vi "SummaryGui.vi"(11 "SeqData":T1={"BeginTS"=timestamp(0 s since 1904-01-01), "EndTS"=timestamp(0 s since 1904-01-01), "State"=enum."Init", "Status.Work"=enum."-", "Status.Process"=enum."-", "Status.Home"=enum."-", "Status.Wabco"=enum."-", "Status.Client"=enum."-", "BreakReason"=enum."-", "BreakSource"=enum."-", "DoorLock"=FALSE, "Status.Prod"=[], "UserAction"={"Stop"=FALSE, "Pause"=FALSE, "Next"=FALSE}, "UserData"={"GuiMode"=enum."Process", "Test"={"IgnoreResults"=FALSE, "IgnoreImages"=FALSE, "ServiceMode"=FALSE}, "ContinueOrder"=FALSE}, "Error"={"status"=FALSE, "code"=0, "source"=""}, "Code"={"Ready"=FALSE, "DoubleOrder"=FALSE, "OrderDone"=FALSE, "AllowSingleSlot"=FALSE, "CheckDM"=FALSE, "ThresholdA"=0, "ThresholdB"=0, "Plate"=enum."Wabco", "ImgPath"=path "", "Variant"={"State"=enum."Init", "ImgPath"=path "", "WabcoPlate"="", "WabcoProduct"="", "ClientProduct"="", "ClientPlate"="", "TotalQuantity"=0, "OrderQuantity"=0, "Serial"=0, "Wabco"={"LaserJob"="", "AdditionalTxt"="037", "FactoryCode"="", "RevID"=0, "ForkID"=0, "FailuresLimit"=0, "GlobalCnt"=0, "Bank"=0, "SerialFormat"=enum."6 dig", "CoordA"={"X"=0.0, "Y"=0.0, "Angle"=0.0}, "CoordB"={"X"=0.0, "Y"=0.0, "Angle"=0.0}, "DMCconfig"=0}, "Client"={"LaserJob"="", "AdditionalTxt"="", "FactoryCode"="037", "RevID"=0, "ForkID"=0, "FailuresLimit"=0, "GlobalCnt"=0, "Bank"=0, "SerialFormat"=enum."6 dig", "CoordA"={"X"=0.0, "Y"=0.0, "Angle"=0.0}, "CoordB"={"X"=0.0, "Y"=0.0, "Angle"=0.0}, "DMCconfig"=0}}}, "Rotations"=0, "ProdIdx"=0, "ProdDone"=[], "PrintedSerials-Wabco"=[], "PrintedSerials-Client"=[], "Counters-Wabco"={"Expected"=0, "Done"=0, "OK"=0, "NOK"=0, "NOKlimit"=0, "Part"=0, "PartOK"=0}, "Counters-Client"={"Expected"=0, "Done"=0, "OK"=0, "NOK"=0, "NOKlimit"=0, "Part"=0, "PartOK"=0}}) -> ()   [LabVIEW 2016]
uses:
  Sequence/Sequence.Data.ctl
  Sequence/Sequence.State.ctl
  Sequence/Sequence.Step.Status.ctl
  Sequence/Sequence.Test.BreakReason.ctl
  Sequence/Sequence.Test.BreakSource.ctl
  Sequence/Sequence.Test.Status.ctl
  Sequence/Sequence.Slot.StatusData.ctl
  Sequence/Sequence.Test.Unload.Status.ctl
  Sequence/Sequence.Prod.StatusData.ctl
  Sequence/Sequence.UserActions.ctl
  Sequence/Sequence.UserData.ctl
  Sequence/Sequence.MainMode.ctl
  MainGui.TestOptions.ctl
  Sequence/Sequence.Code.Sets.ctl
  Sequence/Sequence.PlateType.ctl
  Logger/Logger.Variant.Sets.ctl
  Station/Station.Changeover.State.vi
  Station/Station.Plate.Properties.ctl
  Sequence/Sequence.Code.SerialFormat.ctl
  Drivers/V7310/LowLevel/V7310.Job.Sets.ctl
  Sequence/Sequence.Counters.ctl
  SummaryGui.Action.ctl
  tools/Translator/Translator.Message.ctl
  tools/Translator/Translator.FormatMessage.vi
  Global/ApplicationGlobal.vi
  tools/Translator/Translator.Global.vi
panel:
  out "container removed":bool
  in  "WabcoPlateSelect":bool
  in  "ClientPlateSelect":bool
  out "Total 2":u16 caption="Wymagane"
  out "NOK 2":u16 caption="NOK"
  out "OK 2":u16 caption="OK"
  out "Done 2":u16 caption="Zrobione"
  out "Total":u16 caption="Wymagane"
  out "NOK":u16
  out "OK":u16
  out "Done":u16 caption="Zrobione"
  out "ClientPlate":picture
  out "Client Plate Status":string caption="Status tabliczki Klienta"
  out "WabcoPlate":picture
  out "Wabco Plate Status":string caption="Status tabliczki Wabco"
  out "Message":string
  in  "OKButton":bool
  out "_loop":i32(ring)=4
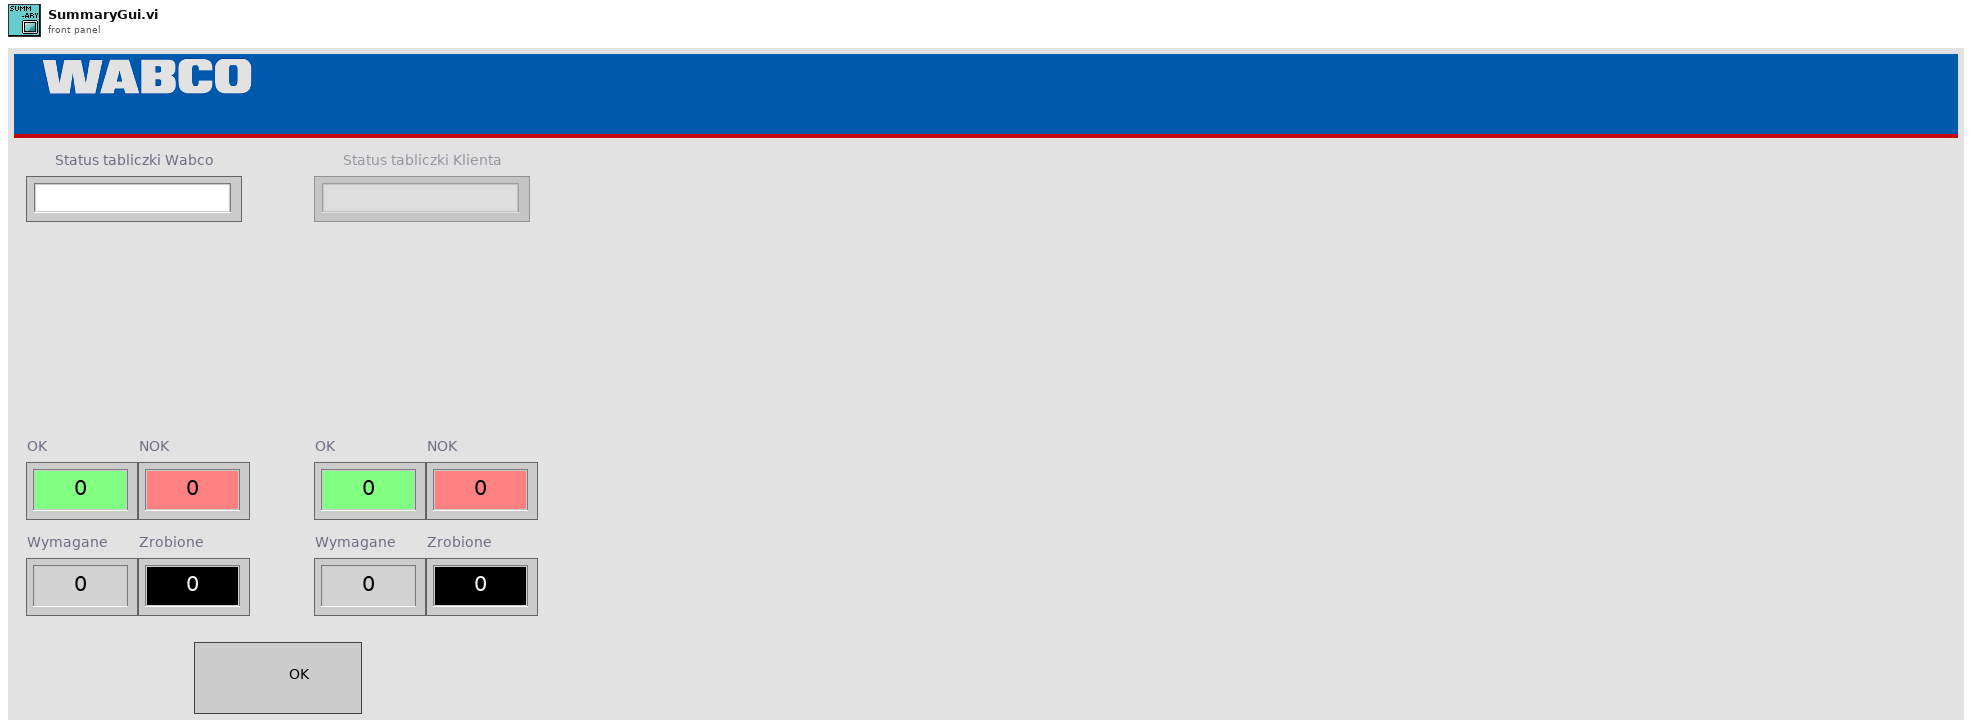
[diagram p1: front panel]
types:
  T1 = typedef "Sequence.Data.ctl" = cluster{"BeginTS":timestamp, "EndTS":timestamp, "State":T2, "Status.Work":T3, "Status.Process":T3, "Status.Home":T3, "Status.Wabco":T3, "Status.Client":T3, "BreakReason":T4, "BreakSource":T5, "DoorLock":bool, "Status.Prod":T6[], "UserAction":T10, "UserData":T11, "Error":errorcluster, "Code":T14, "Rotations":i32, "ProdIdx":i32, "ProdDone":T6[], "PrintedSerials-Wabco":i32[], "PrintedSerials-Client":i32[], "Counters-Wabco":T21, "Counters-Client":T21}
  T2 = typedef "Sequence.State.ctl" = enum16{"Init", "Idle", "Home", "Work", "Run", "Pause"}
  T3 = typedef "Sequence.Step.Status.ctl" = enum16{"-", "Pending", "Running", "Skipped", "Passed", "Failed", "Done", "Error", "Aborted", "Stopped"}
  T4 = typedef "Sequence.Test.BreakReason.ctl" = enum16{"-", "NOK container", "OK container", "Rev empty", "Rev missing", "Rev wrong", "Fork missing", "Fork wrong", "NOK limit", "Unload failure", "Single slot", "Part done", "Err: Prod move work", "Err: Prod move home", "Err: Prod lift work", "Err: Prod lift home", "Err: Prod Arm Work", "Err: Prod Arm NOK", "Err: Prod Arm OK", "Err: Prod NOK suck", "Err: Prod NOK drop", "Err: Prod OK missing", "Err: Prod OK suck", "Err: Prod OK drop"}
  T5 = typedef "Sequence.Test.BreakSource.ctl" = enum16{"-", "A", "B", "A/B"}
  T6 = typedef "Sequence.Test.Status.ctl" = cluster{"Slot":T7, "A":T9, "B":T9}
  T7 = typedef "Sequence.Slot.StatusData.ctl" = cluster{"ID":i32, "Unload":T8, "TS":timestamp, "duration":u32}
  T8 = typedef "Sequence.Test.Unload.Status.ctl" = enum16{"init", "check NOK", "check OK", "wait on NOK", "wait on OK", "wait on Unload", "done"}
  T9 = typedef "Sequence.Prod.StatusData.ctl" = cluster{"status":T3, "pause":T4, "present":bool, "printed":bool, "scanned":bool, "tuned":bool, "removed":bool, "LaserVariables":string[], "ScanerReadOut":string, "path":path, "corners":cluster{"X":i32, "Y":i32}[], "verification":u8}
  T10 = typedef "Sequence.UserActions.ctl" = cluster{"Stop":bool, "Pause":bool, "Next":bool}
  T11 = typedef "Sequence.UserData.ctl" = cluster{"GuiMode":T12, "Test":T13, "ContinueOrder":bool}
  T12 = typedef "Sequence.MainMode.ctl" = enum16{"Process", "Base", "Order", "Manual", "Logs", "Results", "Stats", "DMC Config"}
  T13 = typedef "MainGui.TestOptions.ctl" = cluster{"IgnoreResults":bool, "IgnoreImages":bool, "ServiceMode":bool}
  T14 = typedef "Sequence.Code.Sets.ctl" = cluster{"Ready":bool, "DoubleOrder":bool, "OrderDone":bool, "AllowSingleSlot":bool, "CheckDM":bool, "ThresholdA":u8, "ThresholdB":u8, "Plate":T15, "ImgPath":path, "Variant":T16}
  T15 = typedef "Sequence.PlateType.ctl" = enum16{"Wabco", "Client"}
  T16 = typedef "Logger.Variant.Sets.ctl" = cluster{"State":T17, "ImgPath":path, "WabcoPlate":string, "WabcoProduct":string, "ClientProduct":string, "ClientPlate":string, "TotalQuantity":u16, "OrderQuantity":u16, "Serial":i32, "Wabco":T18, "Client":T18}
  T17 = typedef "Station.Changeover.State.vi" = enum16{"Init", "Scaning", "NOK", "Wait for ack", "Ready"}
  T18 = typedef "Station.Plate.Properties.ctl" = cluster{"LaserJob":string, "AdditionalTxt":string, "FactoryCode":string, "RevID":u8, "ForkID":u8, "FailuresLimit":u16, "GlobalCnt":i32, "Bank":u8, "SerialFormat":T19, "CoordA":T20, "CoordB":T20, "DMCconfig":i32}
  T19 = typedef "Sequence.Code.SerialFormat.ctl" = enum8{"", "6 dig", "7 dig"}
  T20 = typedef "V7310.Job.Sets.ctl" = cluster{"X":dbl, "Y":dbl, "Angle":dbl}
  T21 = typedef "Sequence.Counters.ctl" = cluster{"Expected":u16, "Done":u16, "OK":u16, "NOK":u16, "NOKlimit":u16, "Part":u16, "PartOK":u16}
  T22 = typedef "SummaryGui.Action.ctl" = enum32{"idle", "constructor", "destructor", "--- SummaryGUI ---", "wait for container"}
  T23 = enum8{"Enabled", "Disabled", "Disabled and Grayed Out"}
  T24 = typedef "Translator.Message.ctl" = enum16{"-", "Event confirmed", "Log out", "Log in", "Shutdown", "Cancel", "Start", "Begin time", "End time", "Duration", "Service Mode", "Ignore Results", "Serial Format", "On", "Off", "OK", "NOK", "NOK %s", "Home", "Work", "Close", "Open", "In progress...", "Missing", "Empty", "Hardware failure", "Initial", "Default", "Total", "Out of range", "Free disk space is below 1GB - contact technician", "Error %d >> %s", "Error %d >> %s >> %s", "Msg %d >> %s", "Laser msg %d %s", "Laser cmd error %s %d", "Laser cmd failed %s", "Laser cmd warning %s", "Laser disconnected", "Laser status %s", "Laser already started", "Laser job unkonwn %s", "Laser job missing %s", "Laser job select failure %s", "Unable to start laser printing (%s)", "Unable to stop laser printing (%s)", "Laser marking aborted", "Laser marking timeout", "Unable to reset Laser Interlock (%s)", "Unable to trigger Laser. Laser not ready (%s)", "Laser job '%s' coordinates not configured", "Starting %s", "Quitting %s", "Configured", "Initializing", "Quitting", "Loading", "Loaded %d results", "Loaded %d events", "Running", "Stopped", "Summary", "Laser", "Do you want to continue?", "Do you want to delete the configuration?", "The configuration is being used by an order. Unable to delete!", "Press confirm button", "Station is not based. Do you want to exit?", "Station requires changeover. Do you want to run the test?", "Test options are not set as default. Do you want to continue?", "Formatting of WabcoNo is disabled. Do you want to continue?", "Product not detected. Do you want to continue?", "Product scan failed. Do you want to continue?", "Calibration", "Log out?", "System", "All", "IDLE", "Translating...%s", "Not found", "Alarm %s", "Run", "Skip", "Abort", "Repeat", "Please wait...", "Database disconnected", "Database disconnected - changeover disabled!", "Login to database successful", "Login to database failed: %d; %s", "Unable to check the product status of reference %d - database disconnected", "Unable to set the product status of reference %d - database disconnected", "Variant file backup %s", "Read variant (%s)", "Result", "Station armed!", "Station requires changeover!", "Select reference number...", "EMERGENCY BUTTON - press Control button", "EMERGENCY DOOR - press Control button", "Resetting Emergency...", "Unable to reset safety circuit - Emergency Button pressed", "Unable to reset safety circuit - Emergency Side Door open", "Station not based", "Station based", "Station not empty", "Station basing...", "No order", "Press Start to begin new order", "Scanning new order", "Order NOK. Correct or scan again", "Order OK. Press Accept", "Order ready", "Revolver incorrect", "Fork incorrect", "Revolver missing", "Revolver empty", "Container missing", "Offline results", "Offline statistics", "Updating statistics %.1f %%", "DMC Configurator", "Door open", "Close the front door", "Press start button", "Done. Open the front door", "Running...", "Running...%.1f %%", "Pause %s", "Pause %s. NOK container missing", "Pause %s. OK container missing", "Pause %s. Revolver empty", "Pause %s. Revolver missing", "Pause %s. Revolver incorrect", "Pause %s. Fork missing", "Pause %s. Fork incorrect", "Pause %s. Too many failures", "Pause %s. Unloading failure", "Pause %s. One slot is not working", "Pause %s. Part order is done. Empty OK container", "Pause %s. Unable to move product to slot", "Pause %s. Unable to move back product pusher", "Pause %s. Unable to lift product", "Pause %s. Unable to move back product lifter", "Pause %s. Unable to move product arm to Work", "Pause %s. Unable to move product arm to NOK", "Pause %s. Unable to move product arm to OK", "Pause %s. Unable to unsuck the NOK product", "Pause %s. Unable to drop the NOK product", "Pause %s. Product OK missing", "Pause %s. Unable to unsuck the OK product", "Pause %s. Unable to drop the OK product", "Stopping...", "File '%s' is missing", "File '%s' is broken", "File '%s' is running", "Log file started (%s)", "Log file ended (%s)", "Log file stopped (%s)", "Log file ignored (%s)", "Log file exported (%s)", "Log file export failed (%s)", "Wrong serial number in log file", "Wrong reference number in log file", "Test steps are missing", "%s = %.3f", "Process param '%s' not found in DB", "Process param '%s' wrong order", "Process param '%s' value %.3f out of limits (%.3f; %.3f)", "Step%d param '%s' not found in DB", "Step%d param '%s' wrong order", "Step%d param '%s' value %.3f out of limits (%.3f; %.3f)", "Step%d EV '%s' not found in DB", "Step%d EV '%s' wrong order", "\"%s\" not found in DB", "\"%s\" wrong order", "\"%s\" value %.3f out of limits (%.3f; %.3f)", "\"%s\" not found in software", "Process init (%s)", "Process started", "Process restarted", "Process run", "Process done", "Process done - remove OK container", "Process aborted", "Process aborted at work", "Process aborted at home", "Process error", "Process error at home", "Process error at work", "Process close", "Process pause", "Process continue", "Process door open", "Process door close", "Process pause at slot %s due to %s", "Select plate from the order to process", "Do you want to start the process?", "Do you want to continue the process?", "There is unfinished order. Do you want to put the new order?", "Product %s %d OK", "Product %s %d NOK", "Unable to unload the slot %s. Product missing in the slot", "Unable to unload the slot %s. Product already in the arm", "Unable to accept the product as OK. Product missing in slot %s", "Unable to accept the product as OK. Product could not drop into the container at slot %s", "Unable to accept the product as NOK. Product could not drop into the container at slot %s", "Scan failed. Error %s", "Scan failed. Scanner disconnected", "Scan failed. Wrong Wabco number %d, limit (%d,%d)", "Scan failed. Wrong serial number %d, limit (%d,%d)", "Scan failed. Wrong date %d, limit (%d,%d)", "Scan failed. Wrong product wabco number %d (expected %d)", "Scan failed. Wrong product serial number %d (expected > 0)", "Scan OK %s", "Scan failed. Unable to determine table position (%s)", "Scan failed. Timeout", "Tune failed. Scanner disconnected", "Tune failed. Timeout", "%s = %d", "%s = %d->%d", "Unable to set %s = %.2f - Air Pressure Inside off", "Unable to set digital output '%s' = %d", "Unable to activate air pressure inside - timeout", "Unable to activate air pressure inside - aborted", "Unable to switch on Air Main Valve - Air Pressure Inlet off", "Unable to switch on Air Main Valve - Door open", "Unable to switch off Air Main Valve - timeout", "Unable to switch off Air Main Valve - aborted", "Unable to rotate Table - timeout", "Unable to rotate Table - aborted", "Unable to rotate Table - Product Move not in Home position", "Unable to rotate Table - Air Pressure Inside off", "Unable to rotate Table - Product Lift A not in Home position", "Unable to rotate Table - Product Lift B not in Home position", "Unable to rotate Table - unlock before movement timeout", "Unable to rotate Table - lock after movement timeout", "Unable to move Table Lock to %s position - timeout", "Unable to move Table Lock to %s position - aborted", "Unable to move Table Lock to %s position - Air Pressure Inside off", "Unable to move Table Lock to %s position - Table not in position", "Unable to move Product Lift A to %s position - timeout", "Unable to move Product Lift B to %s position - timeout", "Unable to move Product Lift A to %s position - aborted", "Unable to move Product Lift B to %s position - aborted", "Unable to move Product Lift A to %s position - Air Pressure Inside off", "Unable to move Product Lift B to %s position - Air Pressure Inside off", "Unable to move Product Lift A to %s position - Table not locked", "Unable to move Product Lift B to %s position - Table not locked", "Unable to move Product Lift A to %s position - Product Arm not in Work position", "Unable to move Product Lift B to %s position - Product Arm not in Work position", "Unable to set Product Suction Gripper %s to %s - timeout", "Unable to set Product Suction Gripper %s to %s - aborted", "Unable to set Product Suction Gripper %s to %s - Air Pressure Inside off", "Unable to set Product Suction Gripper %s to %s - Table slot unkown", "Unable to move Product Arm to %s position - timeout", "Unable to move Product Arm to %s position - aborted", "Unable to move Product Arm to %s position - Air Pressure Inside off", "Unable to move Product Arm to %s position - Product Lift A not in Home position", "Unable to move Product Arm to %s position - Product Lift B not in Home position", "Unable to move Product to %s position - timeout", "Unable to move Product to %s position - aborted", "Unable to move Product to %s position - Air Pressure Inside off", "Unable to move Product to %s position - Table not in position"}
  T25 = typedef "FestoCPX.Station.ButtonsState.ctl" = cluster{"Start":bool, "Stop":bool, "Control":bool}
  T26 = typedef "LVPositionTypeDef.ctl" = cluster{"Left":i32, "Top":i32}
  T27 = typedef "imagedata.ctl" = cluster{"image type":i32, "image depth":i32, "image":u8[], "mask":u8[], "colors":u32[], "Rectangle":cluster{"left":i16, "top":i16, "right":i16, "bottom":i16}}
  T28 = typedef "FestoCPX.Station.ProdPresent.ctl" = cluster{"Slot1":cluster{"A":bool, "B":bool}, "Slot2":cluster{"A":bool, "B":bool}, "Slot3":cluster{"A":bool, "B":bool}, "Slot4":cluster{"A":bool, "B":bool}, "Final":cluster{"A":bool, "B":bool}, "OK":cluster{"A":bool, "B":bool}, "Container":cluster{"OK":bool, "NOK":bool}}
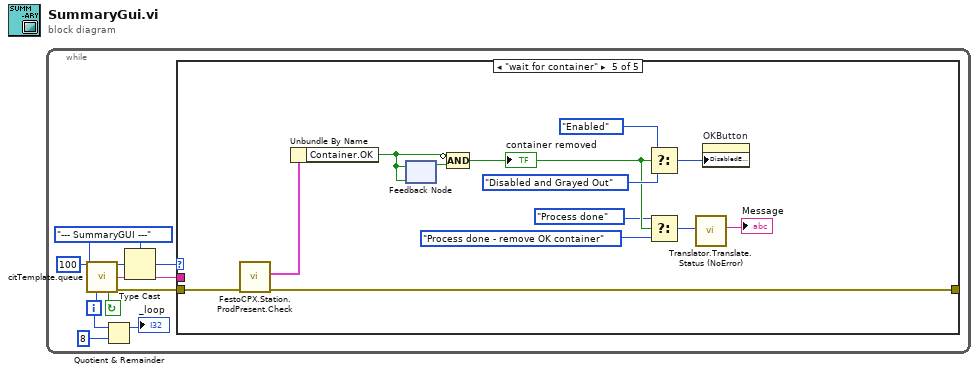
[diagram p0: block diagram]
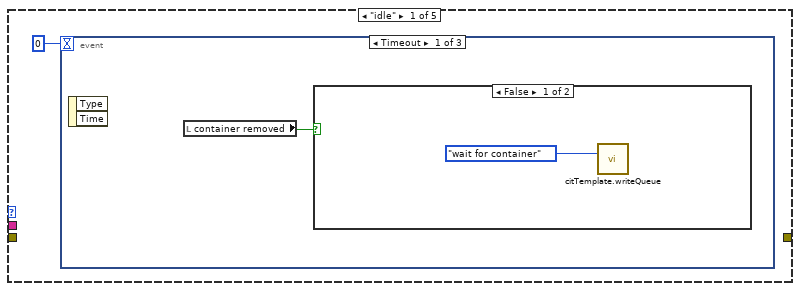
[diagram p2: hidden frame]
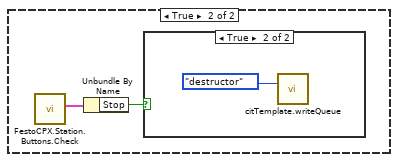
[diagram p3: hidden frame]
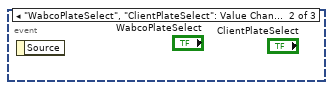
[diagram p5: hidden frame]
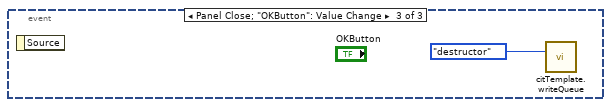
[diagram p6: hidden frame]
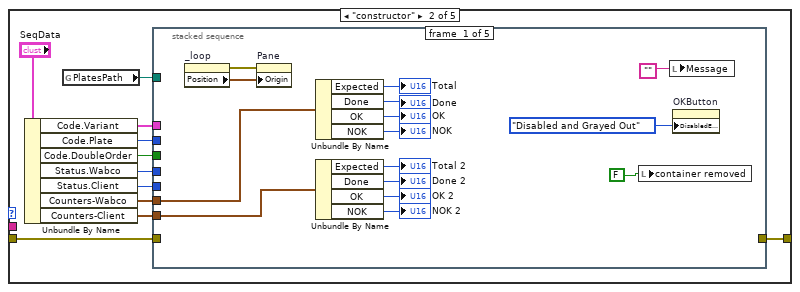
[diagram p7: hidden frame]
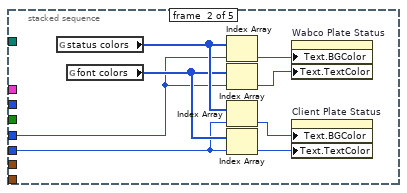
[diagram p8: hidden frame]
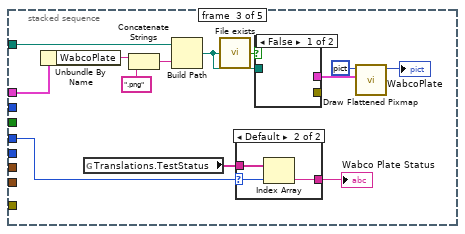
[diagram p9: hidden frame]
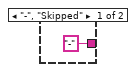
[diagram p10: hidden frame]
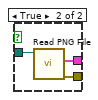
[diagram p11: hidden frame]
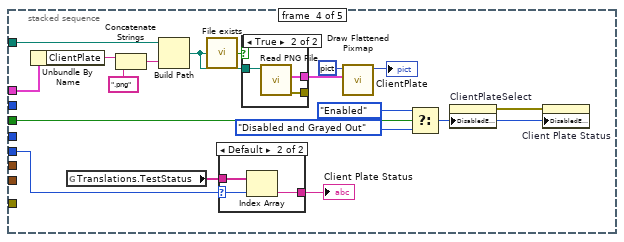
[diagram p12: hidden frame]
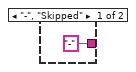
[diagram p13: hidden frame]
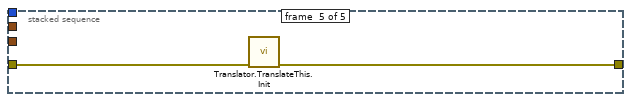
[diagram p15: hidden frame]
diagram:
  n1 = while {
    i -> [w1]
    stop <- w10 continue-if-true
    w4 = SummaryGui.Action."--- SummaryGUI ---" ("Action")
    n2 = call "citTemplate.queue.vi"("ms timeout (250 ms)"=100, "event enum"=w4, "iteration (-1)"=w1) -> ("event out"=w8:u32, "(flatten) data out"=w5:string, "continue"=w10:bool, "error out"=w6:errorcluster)  [unwired: 2 in, 7 out]
    n3 = Quotient & Remainder(x=w1, y=8) -> (x-y*floor(x/y)=→"_loop":i32)  [unwired: 1 out]
    n4 = Type Cast(type=w4, x=w8) -> (*(type *) &x=w7:T22)
    n5 = case shown="\"wait for container\"" w7 {
      tunnel: w6 -> [_ w22 _ _ w109]
      tunnel: w5 -> [_ _ _ _ _]
      tunnel: [_ w21 _ _ w108] -> _
      frame "idle" {
        n6 = event shown="[0] Timeout" {
          selector: _ -> [_ _ _]
          dyn-events: _ -> [_ _ _]
          timeout: 0 -> [_ _ _]
          event Timeout {
            n7 = event-data() -> ()  [unwired: 3 out]
            n8 = local read "container removed"() -> (w12:bool)
            n9 = case shown="False" w12 {
              frame False {
                n10 = call "citTemplate.writeQueue.vi"("event in (if not connected:all statemachine with data event)"=SummaryGui.Action."wait for container" ("Action")) -> ()  [unwired: 14 in, 1 out]
              }
              frame True {
                n11 = call "FestoCPX.Station.Buttons.Check.vi"() -> ("Buttons.State"=w15:T25)  [unwired: 10 in, 1 out]
                n12 = Unbundle By Name(w15) -> ("Stop"=w14:bool)
                n13 = case shown="True" w14 {
                  frame False {
                  }
                  frame True {
                    n14 = call "citTemplate.writeQueue.vi"("event in (if not connected:all statemachine with data event)"=SummaryGui.Action."destructor" ("Action")) -> ()  [unwired: 14 in, 1 out]
                  }
                }
              }
            }
          }
          event "WabcoPlateSelect", "ClientPlateSelect": Value Change {
            n15 = event-data() -> ()  [unwired: 2 out]
          }
          event Panel Close; "OKButton": Value Change {
            n16 = event-data() -> ()  [unwired: 2 out]
            n17 = call "citTemplate.writeQueue.vi"("event in (if not connected:all statemachine with data event)"=SummaryGui.Action."destructor" ("Action")) -> ()  [unwired: 14 in, 1 out]
          }
        }
      }
      frame "constructor" {
        n18 = Unbundle By Name("SeqData") -> ("Code.Variant"=w27:T16, "Code.Plate"=w26:T15, "Code.DoubleOrder"=w23:bool, "Status.Wabco"=w25:T3, "Status.Client"=w24:T3, "Counters-Wabco"=w20:T21, "Counters-Client"=w19:T21)
        n19 = global read "ApplicationGlobal.vi" "PlatesPath"() -> (w28:path)
        n20 = stacked-sequence {
          tunnel: w28 -> [_ _ w56 w82 _]
          tunnel: w27 -> [_ _ w52 w75 _]
          tunnel: w26 -> [_ _ _ _ _]
          tunnel: w25 -> [_ w49 w55 _ _]
          tunnel: w24 -> [_ w46 _ w74 _]
          tunnel: w23 -> [_ _ _ w76 _]
          tunnel: w22 -> [_ _ _ _ w98]
          tunnel: [_ _ _ _ w97] -> w21
          tunnel: w20 -> [w41 _ _ _ _]
          tunnel: w19 -> [w38 _ _ _ _]
          frame #0 {
            n21 = property on="_loop" class="Ring (strict)"() -> (error out=w32:errorcluster, "Position"=w33:T26)  [unwired: 2 in, 1 out]
            n22 = property on="Pane" class="Pane"(error in=w32, "Origin"=w33) -> ()  [unwired: 1 in, 2 out]
            n23 = Unbundle By Name(w41) -> ("Expected"=→"Total":u16, "Done"=→"Done":u16, "OK"=→"OK":u16, "NOK"=→"NOK":u16)
            n24 = Unbundle By Name(w38) -> ("Expected"=→"Total 2":u16, "Done"=→"Done 2":u16, "OK"=→"OK 2":u16, "NOK"=→"NOK 2":u16)
            n25 = local write "container removed"(FALSE ("container removed")) -> ()
            n26 = local write "Message"("") -> ()
            n27 = property on="OKButton" class="Bool"("DisabledEnum"=T23."Disabled and Grayed Out" ("Disabled")) -> ()  [unwired: 2 in, 2 out]
          }
          frame #1 {
            n28 = global read "ApplicationGlobal.vi" "status colors"() -> (w51:u32[])
            n29 = global read "ApplicationGlobal.vi" "font colors"() -> (w50:u32[])
            n30 = Index Array(array=w51, index=w49) -> (element=w48:u32)
            n31 = Index Array(array=w50, index=w49) -> (element=w47:u32)
            n32 = Index Array(array=w51, index=w46) -> (element=w45:u32)
            n33 = Index Array(array=w50, index=w46) -> (element=w44:u32)
            n34 = property on="Wabco Plate Status" class="Str"("Text.BGColor"=w48, "Text.TextColor"=w47) -> ()  [unwired: 2 in, 2 out]
            n35 = property on="Client Plate Status" class="Str"("Text.BGColor"=w45, "Text.TextColor"=w44) -> ()  [unwired: 2 in, 2 out]
          }
          frame #2 {
            n36 = Unbundle By Name(w52) -> ("WabcoPlate"=w61:string)
            n37 = global read "Translator.Global.vi" "Translations.TestStatus"() -> (w53:string[])
            n38 = Concatenate Strings(w61, ".png" ("string")) -> (w62:string)
            n39 = Build Path(base path=w56, name or relative path=w62) -> (appended path=w60:path)
            n40 = call "File exists.vi"("file path"=w60) -> ("exists?"=w59:bool)  [unwired: 4 in]
            n41 = case shown="Default" w55 {
              selector: w55 -> [_ w67]
              tunnel: ["-" ("String") w66] -> w54
              tunnel: w53 -> [_ w68]
              frame "-", "Skipped" {
              }
              frame Default {
                n42 = Index Array(array=w68, index=w67) -> (element=w66:string)
              }
            }
            "Wabco Plate Status" <- w54
            n43 = case shown="False" w59 {
              tunnel: w60 -> [_ w71]
              tunnel: [_ w70] -> w57
              tunnel: [_ w69] -> _
              frame False {
              }
              frame True {
                n44 = call <vilib>:"Read PNG File.vi"("path to PNG file"=w71) -> ("error out"=w69:errorcluster, "image data"=w70:T27)  [unwired: 8 in, 1 out]
              }
            }
            n45 = call <vilib>:"Draw Flattened Pixmap.vi"("image data"=w57, "picture"=picture data[5B]) -> ("new picture"=→"WabcoPlate":picture)  [unwired: 7 in]
          }
          frame #3 {
            n46 = Unbundle By Name(w75) -> ("ClientPlate"=w81:string)
            n47 = global read "Translator.Global.vi" "Translations.TestStatus"() -> (w73:string[])
            n48 = Concatenate Strings(w81, ".png" ("string")) -> (w87:string)
            n49 = Build Path(base path=w82, name or relative path=w87) -> (appended path=w86:path)
            n50 = call "File exists.vi"("file path"=w86) -> ("exists?"=w85:bool)  [unwired: 4 in]
            n51 = case shown="Default" w74 {
              selector: w74 -> [_ w92]
              tunnel: ["-" ("String") w91] -> w72
              tunnel: w73 -> [_ w93]
              frame "-", "Skipped" {
              }
              frame Default {
                n52 = Index Array(array=w93, index=w92) -> (element=w91:string)
              }
            }
            "Client Plate Status" <- w72
            n53 = case shown="True" w85 {
              tunnel: w86 -> [_ w96]
              tunnel: [_ w95] -> w83
              tunnel: [_ w94] -> _
              frame False {
              }
              frame True {
                n54 = call <vilib>:"Read PNG File.vi"("path to PNG file"=w96) -> ("error out"=w94:errorcluster, "image data"=w95:T27)  [unwired: 8 in, 1 out]
              }
            }
            n55 = call <vilib>:"Draw Flattened Pixmap.vi"("image data"=w83, "picture"=picture data[5B]) -> ("new picture"=→"ClientPlate":picture)  [unwired: 7 in]
            n56 = Select(t=T23."Enabled" ("Disabled"), s=w76, f=T23."Disabled and Grayed Out" ("Disabled")) -> (s? t:f=w78:T23)
            n57 = property on="ClientPlateSelect" class="Bool"("DisabledEnum"=w78) -> (error out=w77:errorcluster)  [unwired: 2 in, 1 out]
            n58 = property on="Client Plate Status" class="Str"(error in=w77, "DisabledEnum"=w78) -> ()  [unwired: 1 in, 2 out]
          }
          frame #4 {
            n59 = call "Translator.TranslateThis.Init.vi"("error in"=w98) -> ("error out"=w97:errorcluster)  [unwired: 10 in]
          }
        }
      }
      frame "destructor" {
      }
      frame "--- SummaryGUI ---" {
      }
      frame "wait for container" {
        n60 = call "FestoCPX.Station.ProdPresent.Check.vi"("error in"=w109) -> ("error out"=w108:errorcluster, "Prod Present"=w111:T28)  [unwired: 5 in, 4 out]
        n61 = Unbundle By Name(w111) -> ("Container.OK"=w99:bool)
        n62 = feedback #1(w99) -> (w110:bool)
        n63 = feedback-in #1(w99) -> ()
        n64 = Compound Arithmetic op=AND(invert w99, w110) -> (w103:bool)
        "container removed" <- w103
        n65 = Select(t=T23."Enabled" ("Disabled"), s=w103, f=T23."Disabled and Grayed Out" ("Disabled")) -> (s? t:f=w105:T23)
        n66 = Select(t=Translator.Message."Process done" ("_Msg"), s=w103, f=Translator.Message."Process done - remove OK container" ("_Msg")) -> (s? t:f=w100:T24)
        n67 = call "Translator.Translate.Status (NoError).vi"("msg"=w100) -> ("Translated Msg"=→"Message":string)  [unwired: 10 in]
        n68 = property on="OKButton" class="Bool"("DisabledEnum"=w105) -> ()  [unwired: 2 in, 2 out]
      }
    }
  }
